vi "bats.parser.ip.vi"() -> ()   [LabVIEW 2022 SP3]
uses:
  <vilib>/Platform/TimedLoop/XDataNode/timing_clust.ctl
  <vilib>/Platform/TimedLoop/XDataNode/nitl_modes.ctl
  <vilib>/Platform/TimedLoop/XDataNode/wakeup.ctl
  <vilib>/rvi/Emulation/niFpgaSctlEmulationGetInTimedLoop.vi
  <vilib>/rvi/Emulation/niFpgaEmulationReportErrorSimple.vi
  <vilib>/rvi/Emulation/niFpgaGetClockAttributes.vi
  <vilib>/rvi/Emulation/niFpgaCriticalErrorInLSC.vi
  <vilib>/rvi/Emulation/niFpgaEmulationIsFPGAContextNoSignature.vi
  <vilib>/rvi/errors/niFpgaSetErrorForExecOnDevCompSimple.vi
  <vilib>/rvi/eio/common/nirviEmuReportErrorAndStop.vi
  <vilib>/rvi/DataTransferAndStorage/Container/Common/niFpgaContainerGetUniqueNameForEmu.vi
  <vilib>/rvi/FIFO/Fifo_Resource/nirvififoEmulationSetSize.vi
  <vilib>/rvi/FIFO/Fifo_Resource/nirviFifoEmulationQueueMgr.vi
  <instcachedir>/0/nirviFifoEmulationQueueMgr_E5CAEC123FF24DC58D834DCA3CDAA9B5.lvgen/nirviFifoEmulationQueueMgr_E5CAEC123FF24DC58D834DCA3CDAA9B5_002.vi
  <vilib>/Utility/error.llb/Clear Errors.vi
  <vilib>/rvi/FIFO/Fifo_Resource/nirvififoEmulationCreateLock.vi
  <vilib>/rvi/Emulation/niFpgaProcessEmulError.vi
  <vilib>/rvi/FIFO/Fifo_Resource/nirvififoEmulationObtainLock.vi
  <vilib>/rvi/FIFO/Fifo_Resource/nirvififoEmulationReleaseLock.vi
  <vilib>/rvi/occurrence/nirviWaitOnOccurrenceBase.vi
  <vilib>/rvi/errors/nirviReportUnexpectedCaseInternalError.vi
  <vilib>/rvi/errors/nirviReportUnexpectedCaseInternalError (U32).vi
  <vilib>/Platform/TimedLoop/XDataNode/XDataNode.xnode
  <vilib>/rvi/DataTransferAndStorage/Container/XNode/niFpgaContainer.xnode
  <vilib>/rvi/FIFO/Fifo_Resource/nirvififoEmulationRead.vi
  <vilib>/Platform/TimedLoop/XDataNode/XDNodeRunTimeDep.lvlib
panel:
  in  "conf_valid":bool
  in  "Configuration.In":u64[](array[numeric])=[0, 0]
  out "OrderBook.Command.Valid":bool
  out "Cancelled Quantity (U32)":u32
  out "Executed Quantity (U32)":u32
  out "Price (U64)":u64
  out "Symbol (U64)":u64
  out "Quantity (U32)":u32
  out "Order Id (U64)":u64
  out "Side (U8)":u8
  out "OrderBook Command":T1(ring)
  in  "Ready.for.OrderBook.Command":bool
  out "Ready.for.Udp.Input":bool
  in  "data_valid":bool
  in  "data":u8
  in  "reset":bool
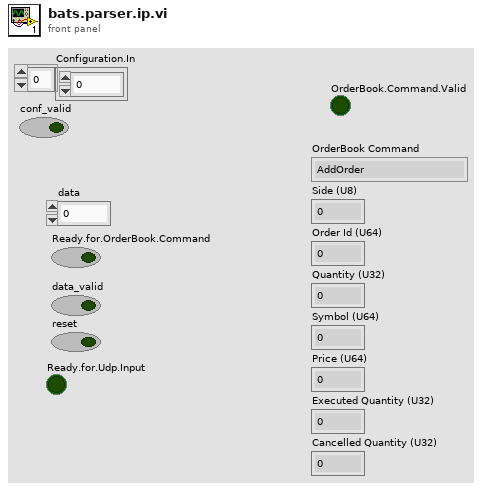
[diagram p1: front panel]
types:
  T1 = enum16{"AddOrder", "OrderExecuted", "ReduceSize", "ModifyOrder", "DeleteOrder"}
  T2 = typedef "XDNodeRunTimeDep.lvlib/timing_clust.ctl" = cluster{"Expected End [f-1]":u64, "Actual End [f-1]":u64, "Finished Late? [f-1]":bool, "Expected End [i-1]":u64, "Actual End [i-1]":u64, "Finished Late? [i-1]":bool, "Expected Start [i]":u64, "Actual Start [i]":u64, "Expected Start [f]":u64, "Actual Start [f]":u64, "Source Name":string, "Structure Name":string, "Period":i64, "Deadline":i64, "Offset":i64, "Start":i64, "Priority":i32, "Timeout":i32, "Mode":T3, "Wakeup Reason":T4, "Error":errorcluster, "Source Type":string, "Secondary Source Type":string, "Global End Time":u64, "Global Start Time":u64, "Frame Duration":u64, "Iteration Duration":u64, "Assigned CPU":i32, "I/O Scan Engine Mode":u32}
  T3 = typedef "XDNodeRunTimeDep.lvlib/nitl_modes.ctl" = enum32{"No Change", "Process missed periods, maintain original phase", "Discard missed periods, maintain original phase", "Process missed periods, ignore original phase", "Discard missed periods, ignore original phase"}
  T4 = typedef "XDNodeRunTimeDep.lvlib/wakeup.ctl" = enum32{"Normal", "Aborted", "Asynchronous wakeup", "Timing source error", "Timed loop error", "Timeout"}
  T5 = cluster{"OrderBook Command.Type":enum16{"AddOrder", "OrderExecuted", "ReduceSize", "ModifyOrder", "DeleteOrder", "Get.All.Orders", "Get.Top"}, "Side (U8)":u8, "Order Id (U64)":u64, "Quantity (U32)":u32, "Symbol (U64)":u64, "Price (U64)":u64, "Executed Quantity (U32)":u32, "Cancelled Quantity (U32)":u32}
  T6 = enum16{"AddOrder", "OrderExecuted", "ReduceSize", "ModifyOrder", "DeleteOrder", "Get.All.Orders", "Get.Top"}
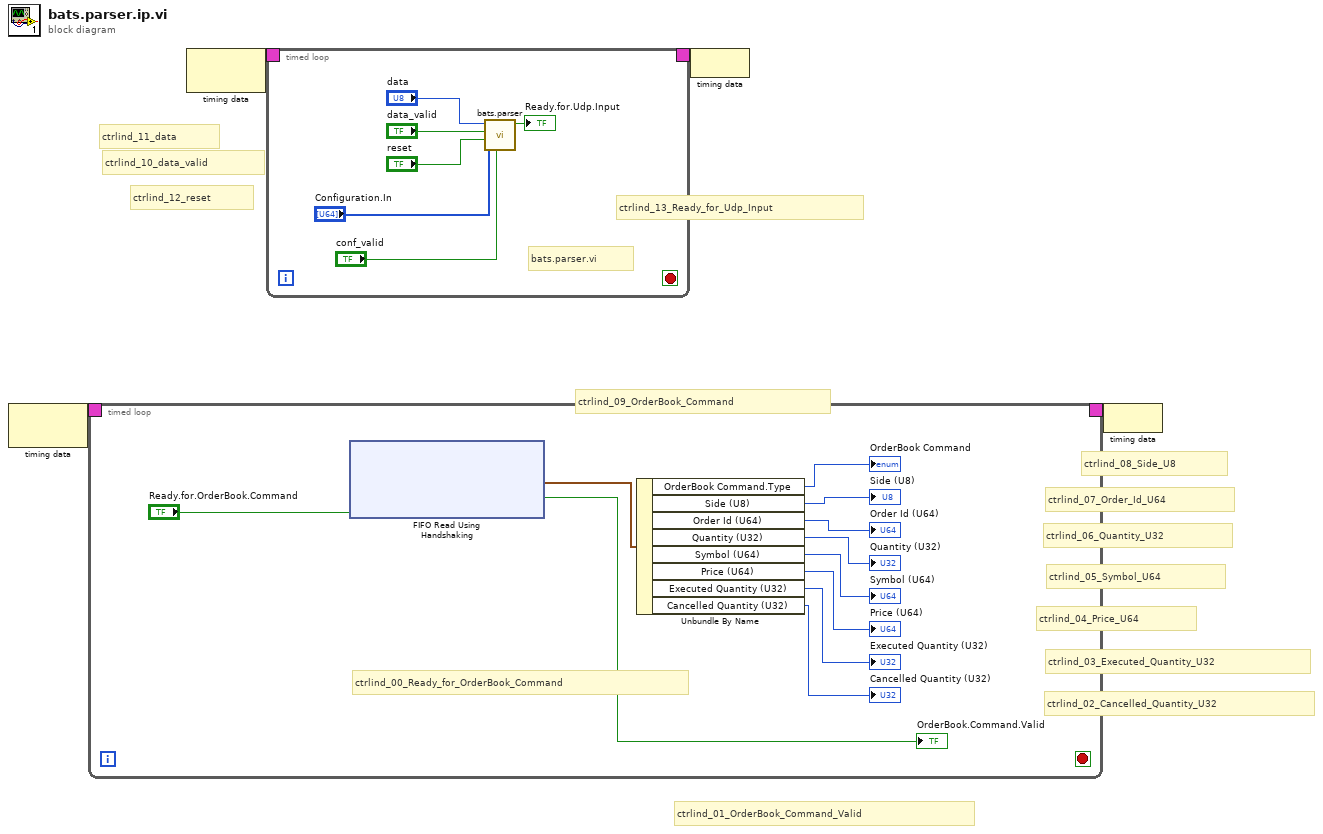
[diagram p0: block diagram]
diagram:
  # "ctrlind_09_OrderBook_Command"
  # "ctrlind_08_Side_U8"
  # "ctrlind_07_Order_Id_U64"
  # "ctrlind_06_Quantity_U32"
  # "ctrlind_05_Symbol_U64"
  # "ctrlind_04_Price_U64"
  # "ctrlind_03_Executed_Quantity_U32"
  # "ctrlind_02_Cancelled_Quantity_U32"
  # "ctrlind_01_OrderBook_Command_Valid"
  # "ctrlind_13_Ready_for_Udp_Input"
  # "ctrlind_11_data"
  # "ctrlind_10_data_valid"
  # "ctrlind_12_reset"
  n1 = node-c288() -> (w2:T2)  [unwired: 1 in]
  n2 = timed-loop {
    timing: w2 -> [_]
    timing-out: [_] -> w1
    stop <- _ stop-if-true
    # "ctrlind_00_Ready_for_OrderBook_Command"
    n3 = xnode ("FIFO Read Using Handshaking")("Ready for Output"="Ready.for.OrderBook.Command") -> ("Element"=w7:T5, "Output Valid"=→"OrderBook.Command.Valid":bool)  [unwired: 1 in, 1 out]
    n4 = Unbundle By Name(w7) -> ("OrderBook Command.Type"=→"OrderBook Command":T6, "Side (U8)"=→"Side (U8)":u8, "Order Id (U64)"=→"Order Id (U64)":u64, "Quantity (U32)"=→"Quantity (U32)":u32, "Symbol (U64)"=→"Symbol (U64)":u64, "Price (U64)"=→"Price (U64)":u64, "Executed Quantity (U32)"=→"Executed Quantity (U32)":u32, "Cancelled Quantity (U32)"=→"Cancelled Quantity (U32)":u32)
  }
  n5 = node-c288() -> (w4:T2)  [unwired: 1 in]
  n6 = timed-loop {
    timing: w4 -> [_]
    timing-out: [_] -> w3
    stop <- _ stop-if-true
    # "bats.parser.vi"
    n7 = call "bats.parser.vi"("conf_valid"="conf_valid", "Configuration.In"="Configuration.In", "reset"="reset", "data_valid"="data_valid", "data"="data") -> ("Ready.for.Udp.Input"=→"Ready.for.Udp.Input":bool)  [unwired: 5 in, 1 out]
  }
  n8 = node-c288(w3) -> ()
  n9 = node-c288(w1) -> ()
